vi "ReadTree.vi"(8 "error in":errorcluster, 10 "root":T1, 11 "repository in":refnum<class "NISE_CEF_Repository.lvclass">) -> (0 "error out":errorcluster, 3 "repository out":refnum<class "NISE_CEF_Repository.lvclass">)   [LabVIEW 2013, in "NISE_CEF_Repository.lvclass"]
doc: "Transfers information between the repo and the tree control nodes. This should be called before custom views are launched or saving to disk."
uses:
  NISE_CEF_Repository.lvclass
  Node/NodeRef.ctl
  Node/NISE_CEF_Node.lvclass
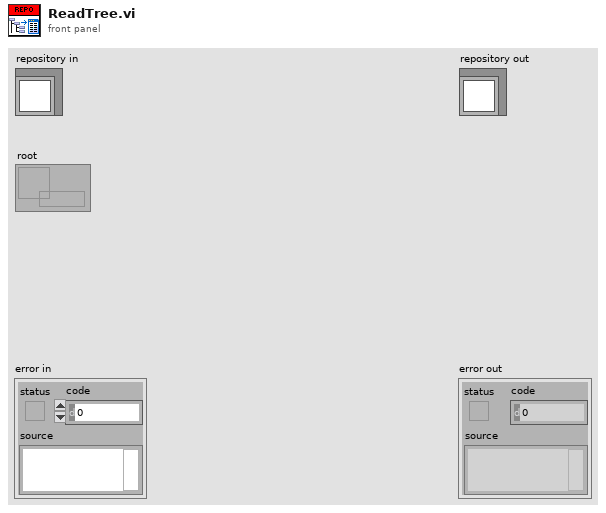
[diagram p1: front panel]
types:
  T1 = typedef "NISE_CEF_Node.lvclass/NodeRef.ctl" = refnum<data-value>
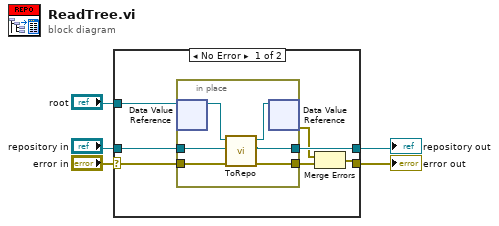
[diagram p0: block diagram]
diagram:
  n1 = case shown="No Error" "error in" {
    selector: "error in" -> [w9 w20]
    tunnel: [w7 w20] -> w4
    tunnel: [w11 w19] -> w2
    tunnel: "repository in" -> [w12 w19]
    tunnel: "root" -> [w10 _]
    frame No Error {
      n2 = in-place {
        in-place-border: w9 -> [w16]
        in-place-border: [w15] -> w8
        in-place-border: w12 -> [w14]
        in-place-border: [w13] -> w11
        n3 = in-place-dvr #1(w10) -> (w18:refnum<class "NISE_CEF_Node.lvclass">)  [unwired: 1 out]
        n4 = call-dynamic "ToRepo.vi"("error in"=w16, "repository in"=w14, "node in"=w18) -> ("error out"=w15:errorcluster, "repository out"=w13:refnum<class "NISE_CEF_Repository.lvclass">, "node out"=w17:refnum<class "NISE_CEF_Node.lvclass">)  [unwired: 6 in]
        n5 = in-place-dvr #1(w17) -> (w6:errorcluster)  [unwired: 1 out]
      }
      n6 = Merge Errors(w6, w8) -> (w7:errorcluster)
    }
    frame Error {
    }
  }
  "error out" <- w4
  "repository out" <- w2
